vi "ModifyUser.vi"(9 "产品型号":refnum<vi>) -> ()   [LabVIEW 2013]
doc: "This VI is the solution to Exercise 3-1 of the LabVIEW Basics II course.\n\nThis VI will accept a user name and password, and after the OK button is pressed, verify if the information is valid using the Verify Information subVI. The name and password controls are initialized to empty strings and the Key Focus attribute of the Login Name control is set to TRUE.\n\nYou will use this VI in Application Exercise.vi (Exercise 5-1) as your login screen."
uses:
  GlobValue.vi
  <vilib>/Utility/config.llb/Write Key (String).vi
  <vilib>/Utility/config.llb/NI_LVConfig.lvlib
panel:
  out "error out":errorcluster caption="错误输出"
  in  "error in":errorcluster
  in  "Cancel":bool
  in  "save":bool
  in  "Password":string
  in  "用户名":string
  # "修改用户名和密码"
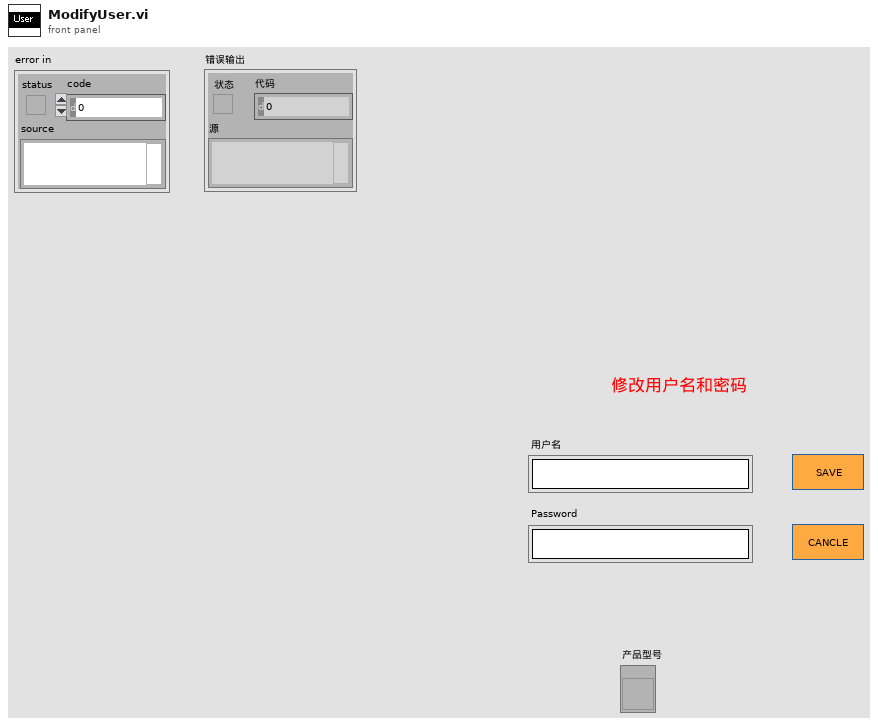
[diagram p1: front panel]
types:
  T1 = typedef "NI_LVConfig.lvlib/Config Data RefNum.ctl" = refnum<k1>
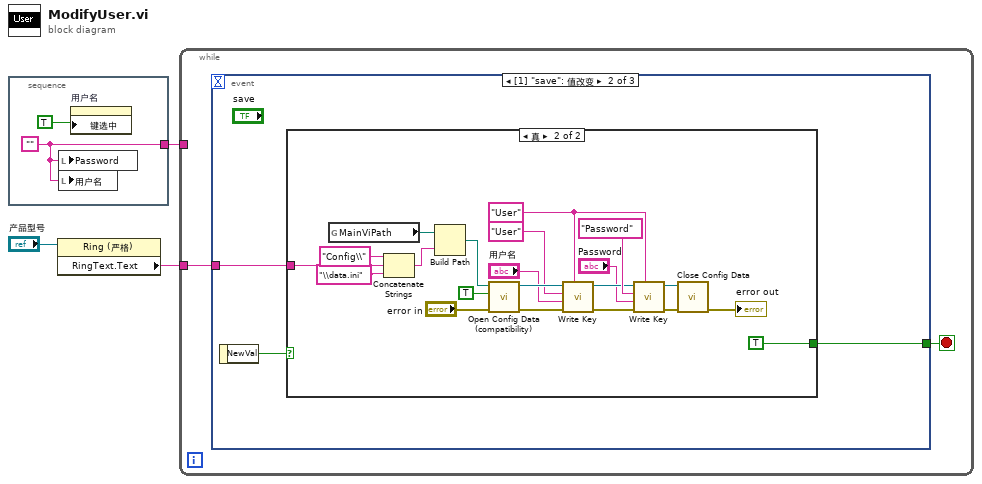
[diagram p0: block diagram]
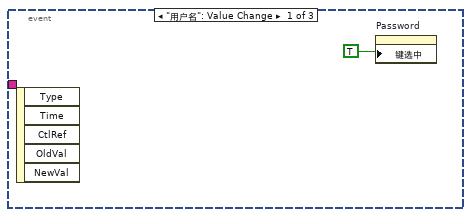
[diagram p2: hidden frame]
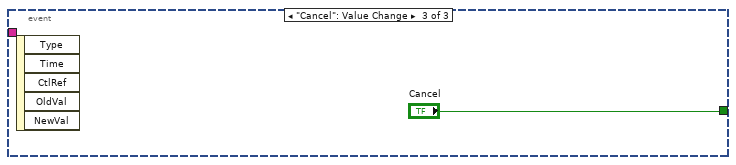
[diagram p4: hidden frame]
diagram:
  n1 = stacked-sequence {
    tunnel: [w4] -> w3
    frame #0 {
      w4 = ""
      n2 = local write "Password"(w4) -> ()
      n3 = local write "用户名"(w4) -> ()
      n4 = property on="用户名" class="Str"("键选中"=TRUE ("Key Focus")) -> ()  [unwired: 2 in, 2 out]
    }
  }
  n5 = property class="Ring (严格)"(reference="产品型号") -> ("RingText.Text"=w1:string)  [unwired: 1 in, 2 out]
  n6 = while {
    tunnel: w3 -> [_]
    tunnel: w1 -> [w6]
    stop <- w7 stop-if-true
    n7 = event shown="[1] \"save\": 值改变" {
      selector: _ -> [_ _ _]
      dyn-events: _ -> [_ _ _]
      timeout: _ -> [_ _ _]
      tunnel: [_ w10 "Cancel"] -> w7
      tunnel: w6 -> [_ w9 _]
      event "用户名": Value Change {
        n8 = event-data() -> ()  [unwired: 6 out]
        n9 = property on="Password" class="Str"("键选中"=TRUE ("Key Focus")) -> ()  [unwired: 2 in, 2 out]
      }
      event "save": Value Change {
        n10 = event-data() -> ("NewVal"=w11:bool)  [unwired: 1 out]
        n11 = case shown="真" w11 {
          tunnel: [_ TRUE] -> w10
          tunnel: w9 -> [_ w14]
          frame False {
          }
          frame True {
            w28 = "User" ("ModelName")
            n12 = global read "GlobValue.vi" "MainViPath"() -> (w17:path)
            n13 = Concatenate Strings("Config\\" ("名称或相对路径"), w14, "\\data.ini") -> (w12:string)
            n14 = Build Path(base path=w17, name or relative path=w12) -> (appended path=w23:path)
            n15 = call <vilib>:"Open Config Data (compatibility).vi"("error in (no error)"="error in", "create file if necessary (T)"=TRUE, "configuration file path"=w23) -> ("error out"=w32:errorcluster, "refnum"=w30:T1)  [unwired: 6 in, 1 out]
            n16 = call-poly <vilib>:"Write Key.vi"("section"=w28, "error in (no error)"=w32, "value"="用户名", "key"="User", "refnum"=w30) -> ("error out"=w27:errorcluster, "refnum out"=w26:T1)  [unwired: 1 in, 4 out]
            n17 = call-poly <vilib>:"Write Key.vi"("section"=w28, "error in (no error)"=w27, "value"="Password", "key"="Password", "refnum"=w26) -> ("error out"=w16:errorcluster, "refnum out"=w31:T1)  [unwired: 1 in, 4 out]
            n18 = call <vilib>:"Close Config Data.vi"("error in (no error)"=w16, "refnum"=w31) -> ("error out"=→"error out":errorcluster)  [unwired: 1 in, 8 out]
          }
        }
      }
      event "Cancel": Value Change {
        n19 = event-data() -> ()  [unwired: 6 out]
      }
    }
  }
